vi "Dialog_about_program_v (SubVI).vi"(11 "Param":T1={"Версия:"="1.2.0", "Наименование ПО:"="SNK3.exe", "Год выпуска:"="2024", "Производитель:"="АО \"НИКИЭТ\"", "MD5"="", "Наименование ПО полное:"="SNK3.exe", "Build"="2.0.0"}) -> ()   [LabVIEW 2017]
panel:
  out "String Indicator":string
  out "MD5":string caption="Цифровой идентификатор (MD5)"
  out "Производитель:":string
  out "Год выпуска основного ПО:":string
  out "Наименование основного ПО:":string
  out "Версия основного ПО:":string
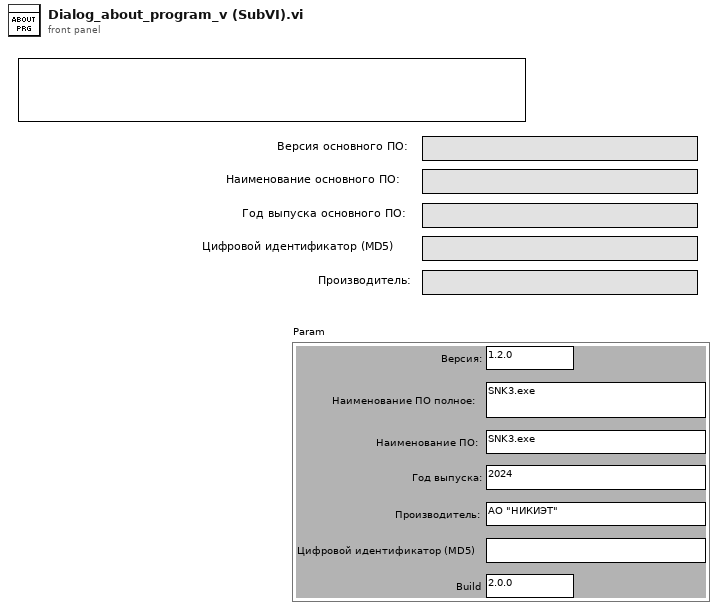
[diagram p1: front panel]
types:
  T1 = cluster{"Версия:":string, "Наименование ПО:":string, "Год выпуска:":string, "Производитель:":string, "MD5":string, "Наименование ПО полное:":string, "Build":string}
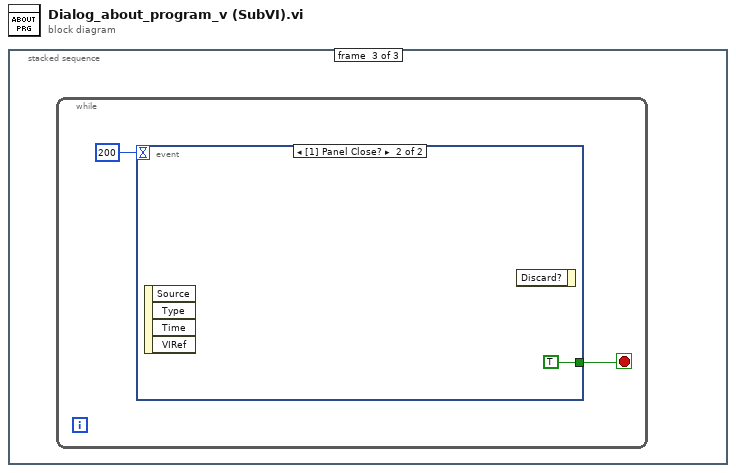
[diagram p0: block diagram]
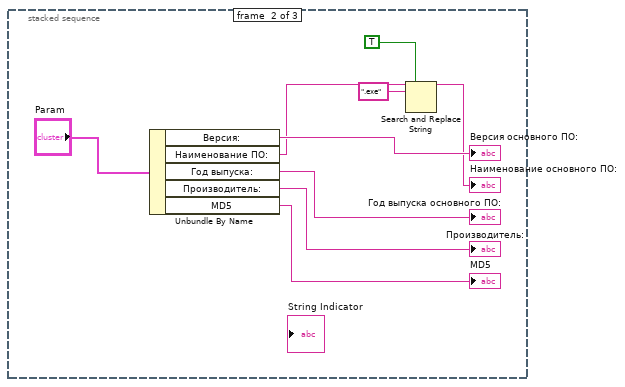
[diagram p3: hidden frame]
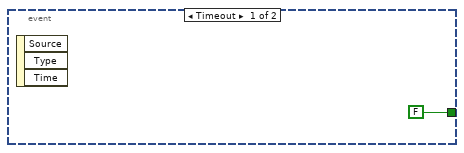
[diagram p4: hidden frame]
diagram:
  n1 = stacked-sequence {
    frame #0 {
    }
    frame #1 {
      n2 = Unbundle By Name("Param") -> ("Версия:"=→"Версия основного ПО:":string, "Наименование ПО:"=w2:string, "Год выпуска:"=→"Год выпуска основного ПО:":string, "Производитель:"=→"Производитель:":string, "MD5"=→"MD5":string)
      n3 = Search and Replace String(replace all?=TRUE ("replace all? (F)"), input string=w2, search string=".exe") -> (result string=→"Наименование основного ПО:":string)  [unwired: 5 in, 3 out]
    }
    frame #2 {
      n4 = while {
        stop <- w10 stop-if-true
        n5 = event shown="[1] Panel Close?" {
          selector: _ -> [_ _]
          dyn-events: _ -> [_ _]
          timeout: 200 -> [_ _]
          tunnel: [FALSE TRUE] -> w10
          event Timeout {
            n6 = event-data() -> ()  [unwired: 1 in, 3 out]
          }
          event Panel Close? {
            n7 = event-data() -> ()  [unwired: 1 in, 4 out]
            n8 = event-data() -> ()  [unwired: 2 in, 1 out]
          }
        }
      }
    }
  }
